vi "Create Tick Lines.vi"(0 "Grid Plane Visible":T1, 1 "Major Ticks":u16, 2 "Minor Ticks":u16, 3 "Major Color":u32(colorbox), 4 "Minor Color":u32(colorbox), 5 "error in (no error)":errorcluster, 6 "Tick Cluster Array":T2, 7 "Draw Major":bool, 8 "Range":cluster{"Max":sgl, "Min":sgl}, 9 "Draw Minor":bool, 10 "Axis":enum16{"X-Axis", "Y-Axis", "Z-Axis"}(ring), 11 "Inverted?":bool, 13 "Logarithm?":bool) -> (14 "Axis Tick Object Out":refnum<vi>, 19 "error out":errorcluster)   [LabVIEW 2020, in "3D Plot.lvclass"]
uses:
  <vilib>/Math Plots/3D Math Plots/3D Plot/3D Plot/3D Plot.lvclass
  <vilib>/Math Plots/3D Math Plots/3D Plot/3D Plot/Typedef/Tick Array.ctl
  <vilib>/picture/3D Picture Control/Object/Create Object (name).vi
  <vilib>/picture/3D Picture Control/NI_3D Picture Control.lvlib
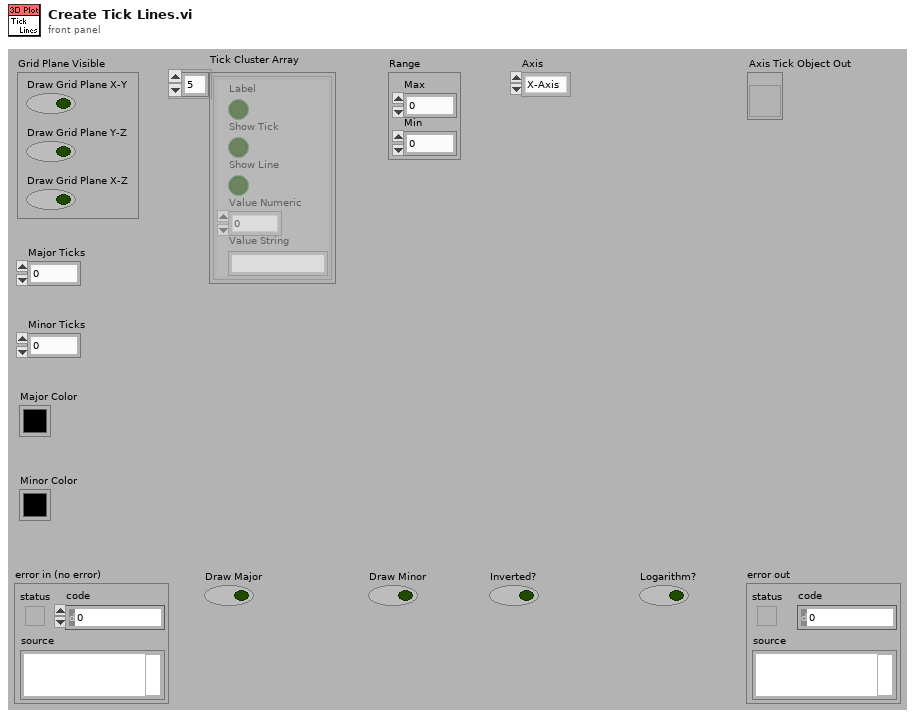
[diagram p1: front panel]
types:
  T1 = cluster{"Draw Grid Plane X-Y":bool, "Draw Grid Plane Y-Z":bool, "Draw Grid Plane X-Z":bool}
  T2 = typedef "3D Plot.lvclass/Tick Array.ctl" = cluster{"Label":bool, "Show Tick":bool, "Show Line":bool, "Value Numeric":sgl, "Value String":string}[]
  T3 = enum16{"Overall", "Per Primitive", "Per Vertex", "Binding Off"}
  T4 = enum16{"Points", "Lines", "Line Strip", "Line Loop", "Triangles", "Triangle Strip", "Triangle Fan", "Quads", "Quad Strip", "Polygon"}
  T5 = cluster{"length":sgl, "length":sgl, "length":sgl}
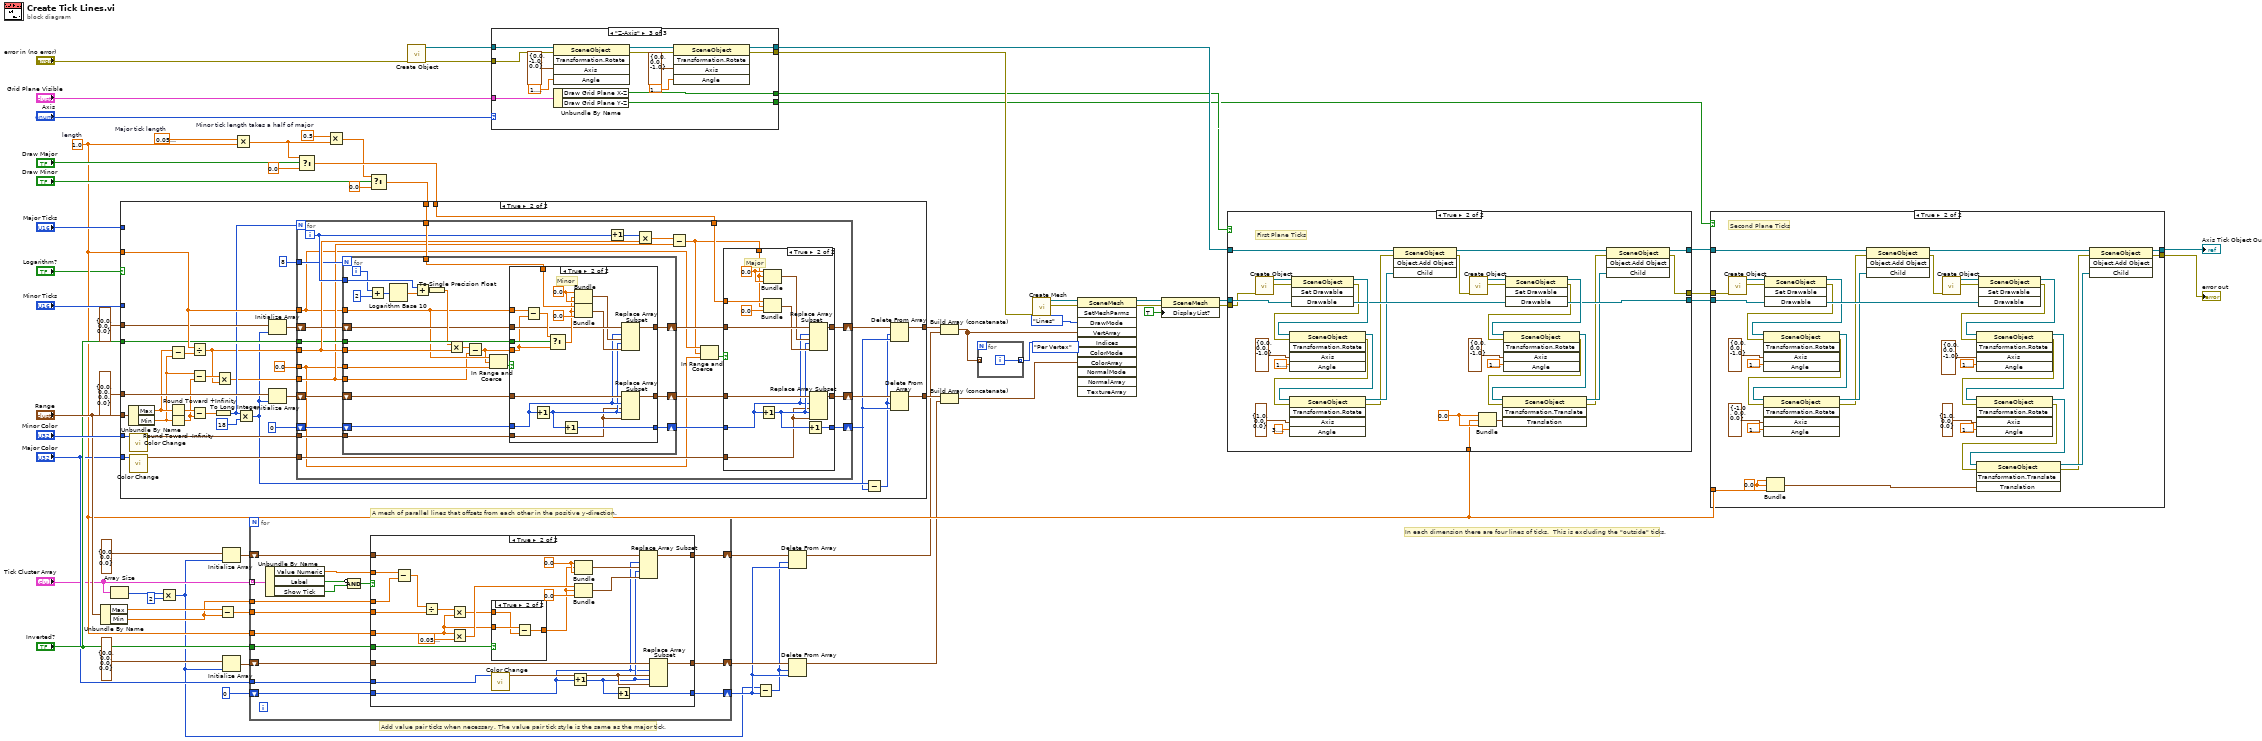
[diagram p0: block diagram]
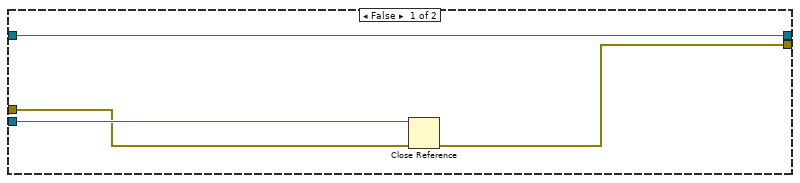
[diagram p2: hidden frame]
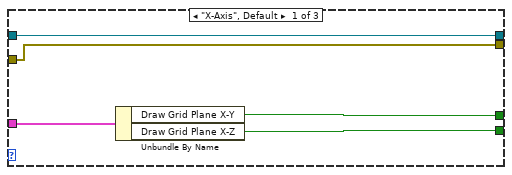
[diagram p4: hidden frame]
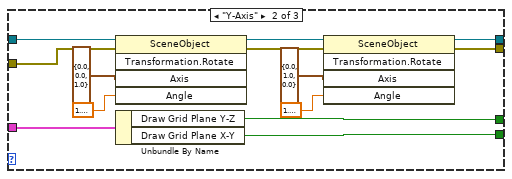
[diagram p5: hidden frame]
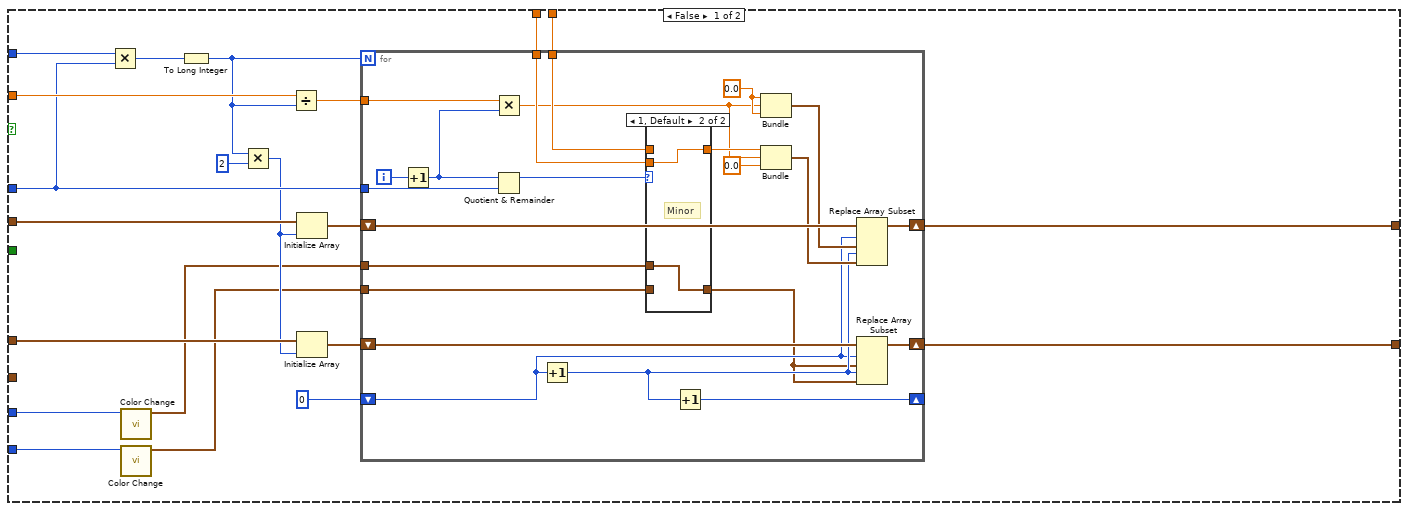
[diagram p6: hidden frame]
diagram:
  w57 = sgl 1.0  # length
  w39 = sgl 0.5  # Minor tick length takes a half of major
  w38 = sgl 0.05  # Major tick length
  # "Add value pair ticks when necessary. The value pair tick style is the same as the major tick."
  # "In each dimension there are four lines of ticks.  This is excluding the \"outside\" ticks."
  # "A mesh of parallel lines that offsets from each other in the positive y-direction."
  n1 = Unbundle By Name("Range") -> ("Max"=w25:sgl, "Min"=w24:sgl)
  n2 = Array Size(array="Tick Cluster Array") -> (size(s)=w4:i32)
  n3 = Multiply(x=w4, y=2 ("x")) -> (x*y=w2:i32)
  n4 = Subtract(x=w25, y=w24) -> (x-y=w35:sgl)
  n5 = Initialize Array(cluster{"X":sgl, "Y":sgl, "Z":sgl} {"X"=0.0, "Y"=0.0, "Z"=0.0} ("3D Point"), w2) -> (w13:cluster{"X":sgl, "Y":sgl, "Z":sgl}[])
  n6 = Initialize Array(cluster{"R":sgl, "G":sgl, "B":sgl, "A":sgl} {"R"=0.0, "G"=0.0, "B"=0.0, "A"=0.0} ("RGBA"), w2) -> (w11:cluster{"R":sgl, "G":sgl, "B":sgl, "A":sgl}[])
  n7 = Multiply(x=w38, y=w57) -> (x*y=w45:sgl)
  n8 = for {
    tunnel: "Tick Cluster Array" -> [w82] mode=indexing
    tunnel: w57 -> [w75]
    tunnel: w35 -> [w77]
    tunnel: w24 -> [w76]
    tunnel: "Inverted?" -> [w74]
    tunnel: "Major Color" -> [w73]
    shift-right: [w72] -> w7
    shift-left: w11 -> [w71]
    shift-right: [w70] -> w9
    shift-left: w13 -> [w69]
    shift-right: [w67] -> w5
    shift-left: 0 -> [w68]
    n9 = Unbundle By Name(w82) -> ("Value Numeric"=w78:sgl, "Label"=w81:bool, "Show Tick"=w80:bool)
    n10 = Compound Arithmetic op=AND(invert w81, w80) -> (w79:bool)
    n11 = case shown="True" w79 {
      tunnel: w78 -> [_ w104]
      tunnel: w77 -> [_ w108]
      tunnel: w76 -> [_ w107]
      tunnel: w75 -> [_ w97]
      tunnel: w74 -> [_ w99]
      tunnel: w73 -> [_ w102]
      tunnel: [w84 w89] -> w72
      tunnel: w71 -> [w84 w90]
      tunnel: [w85 w91] -> w70
      tunnel: w69 -> [w85 w94]
      tunnel: w68 -> [w83 w86]
      tunnel: [w83 w95] -> w67
      frame False {
      }
      frame True {
        w100 = sgl 0.0
        n12 = Subtract(x=w104, y=w107) -> (x-y=w106:sgl)
        n13 = Divide(x=w106, y=w108) -> (x/y=w105:sgl)
        n14 = Multiply(x=w105, y=w97) -> (x*y=w98:sgl)
        n15 = Multiply(x=w97, y=sgl 0.05 ("x")) -> (x*y=w103:sgl)
        n16 = case shown="True" w99 {
          tunnel: w98 -> [w110 w112]
          tunnel: w97 -> [_ w113]
          tunnel: [w110 w111] -> w96
          frame False {
          }
          frame True {
            n17 = Subtract(x=w113, y=w112) -> (x-y=w111:sgl)
          }
        }
        n18 = call <vilib>:"Color Change.vi"("Color"=w102) -> ("RGBA"=w88:cluster{"R":sgl, "G":sgl, "B":sgl, "A":sgl})  [unwired: 1 in, 9 out]
        n19 = Increment(x=w86) -> (x+1=w87:i32)
        n20 = Bundle(w100, w96, w100) -> (w93:cluster{sgl, sgl, sgl})  [unwired: 1 out]
        n21 = Bundle(w103, w96, sgl 0.0) -> (w92:cluster{sgl, sgl, sgl})  [unwired: 1 out]
        n22 = Increment(x=w87) -> (x+1=w95:i32)
        n23 = Replace Array Subset(array=w94, new element #1=w93, index #1=w86, new element #2=w92, index #2=w87) -> (w91:cluster{"X":sgl, "Y":sgl, "Z":sgl}[])
        n24 = Replace Array Subset(array=w90, new element #1=w88, index #1=w86, new element #2=w88, index #2=w87) -> (w89:cluster{"R":sgl, "G":sgl, "B":sgl, "A":sgl}[])
      }
    }
  }
  n25 = Select(t=w45, s="Draw Major", f=sgl 0.0) -> (s? t:f=w50:sgl)
  n26 = Multiply(x=w39, y=w45) -> (x*y=w48:sgl)
  n27 = Select(t=w48, s="Draw Minor", f=sgl 0.0) -> (s? t:f=w47:sgl)
  n28 = case shown="True" "Logarithm?" {
    tunnel: w50 -> [w134 w192]
    tunnel: w47 -> [w133 w193]
    tunnel: "Minor Color" -> [w115 w166]
    tunnel: cluster{"R":sgl, "G":sgl, "B":sgl, "A":sgl} {"R"=0.0, "G"=0.0, "B"=0.0, "A"=0.0} ("RGBA") -> [w125 w187]
    tunnel: "Major Color" -> [w117 w168]
    tunnel: w57 -> [w131 w191]
    tunnel: [w130 w171] -> w34
    tunnel: [w129 w169] -> w33
    tunnel: "Minor Ticks" -> [w128 _]
    tunnel: "Major Ticks" -> [w127 _]
    tunnel: "Range" -> [_ w195]
    tunnel: "Inverted?" -> [_ w190]
    tunnel: cluster{"X":sgl, "Y":sgl, "Z":sgl} {"X"=0.0, "Y"=0.0, "Z"=0.0} ("3D Point") -> [w126 w189]
    frame False {
      n29 = Multiply(x=w127, y=w128) -> (x*y=w122:u16)
      n30 = call <vilib>:"Color Change.vi"("Color"=w115) -> ("RGBA"=w114:cluster{"R":sgl, "G":sgl, "B":sgl, "A":sgl})  [unwired: 1 in, 9 out]
      n31 = call <vilib>:"Color Change.vi"("Color"=w117) -> ("RGBA"=w116:cluster{"R":sgl, "G":sgl, "B":sgl, "A":sgl})  [unwired: 1 in, 9 out]
      n32 = To Long Integer(number=w122) -> (32bit integer=w118:i32)
      n33 = Multiply(x=w118, y=2) -> (x*y=w120:i32)
      n34 = Divide(x=w131, y=w118) -> (x/y=w132:sgl)
      n35 = Initialize Array(w126, w120) -> (w123:cluster{"X":sgl, "Y":sgl, "Z":sgl}[])
      n36 = Initialize Array(w125, w120) -> (w124:cluster{"R":sgl, "G":sgl, "B":sgl, "A":sgl}[])
      n37 = for {
        N: w118 -> [_]
        tunnel: w132 -> [w157]
        tunnel: w128 -> [w156]
        tunnel: w134 -> [w155]
        tunnel: w133 -> [w154]
        shift-right: [w142] -> w130
        shift-left: w123 -> [w145]
        tunnel: w116 -> [w149]
        tunnel: w114 -> [w148]
        shift-right: [w140] -> w129
        shift-left: w124 -> [w141]
        shift-right: [w139] -> _
        shift-left: 0 ("y") -> [w137]
        i -> [w147]
        w146 = sgl 0.0
        n38 = Increment(x=w147) -> (x+1=w150:i32)
        n39 = Multiply(x=w157, y=w150) -> (x*y=w136:sgl)
        n40 = Quotient & Remainder(x=w150, y=w156) -> (x-y*floor(x/y)=w153:i32)  [unwired: 1 out]
        n41 = Increment(x=w137) -> (x+1=w138:i32)
        n42 = case shown="1, Default" w153 {
          tunnel: w155 -> [w159 _]
          tunnel: w154 -> [_ w161]
          tunnel: [w159 w161] -> w151
          tunnel: w149 -> [w158 _]
          tunnel: w148 -> [_ w160]
          tunnel: [w158 w160] -> w135
          frame 0 {
            # "Major"
          }
          frame 1, Default {
            # "Minor"
          }
        }
        n43 = Increment(x=w138) -> (x+1=w139:i32)
        n44 = Bundle(w146, w136, w146) -> (w144:cluster{sgl, sgl, sgl})  [unwired: 1 out]
        n45 = Bundle("f"=w151, w136, sgl 0.0) -> (w143:cluster{"f":sgl, sgl, sgl})  [unwired: 1 out]
        n46 = Replace Array Subset(array=w145, new element #1=w144, index #1=w137, new element #2=w143, index #2=w138) -> (w142:cluster{"X":sgl, "Y":sgl, "Z":sgl}[])
        n47 = Replace Array Subset(array=w141, new element #1=w135, index #1=w137, new element #2=w135, index #2=w138) -> (w140:cluster{"R":sgl, "G":sgl, "B":sgl, "A":sgl}[])
      }
    }
    frame True {
      n48 = Unbundle By Name(w195) -> ("Max"=w180:sgl, "Min"=w178:sgl)
      n49 = call <vilib>:"Color Change.vi"("Color"=w166) -> ("RGBA"=w165:cluster{"R":sgl, "G":sgl, "B":sgl, "A":sgl})  [unwired: 1 in, 9 out]
      n50 = call <vilib>:"Color Change.vi"("Color"=w168) -> ("RGBA"=w167:cluster{"R":sgl, "G":sgl, "B":sgl, "A":sgl})  [unwired: 1 in, 9 out]
      n51 = Subtract(x=w180, y=w178) -> (x-y=w179:sgl)
      n52 = Round Toward +Infinity(x=w180) -> (ceil(x): smallest int >= x=w181:sgl)
      n53 = Round Toward -Infinity(1:w178) -> (0:w177:sgl)
      n54 = Divide(x=w191, y=w179) -> (x/y=w175:sgl)
      n55 = Subtract(x=w178, y=w177) -> (x-y=w176:sgl)
      n56 = Subtract(x=w181, y=w177) -> (x-y=w194:sgl)
      n57 = To Long Integer(number=w194) -> (32bit integer=w182:i32)
      n58 = Multiply(x=w176, y=w175) -> (x*y=w174:sgl)
      n59 = Multiply(x=w182, y=18 ("x")) -> (x*y=w164:i32)
      n60 = Initialize Array(w189, w164) -> (w188:cluster{"X":sgl, "Y":sgl, "Z":sgl}[])
      n61 = Initialize Array(w187, w164) -> (w186:cluster{"R":sgl, "G":sgl, "B":sgl, "A":sgl}[])
      n62 = for {
        N: w182 -> [_]
        shift-right: [w212] -> w170
        shift-left: w186 -> [w218]
        shift-right: [w214] -> w172
        shift-left: w188 -> [w219]
        tunnel: w175 -> [w208]
        tunnel: w193 -> [w217]
        tunnel: w165 -> [w216]
        tunnel: w192 -> [w211]
        tunnel: w167 -> [w202]
        tunnel: w191 -> [w199]
        tunnel: w190 -> [w207]
        shift-right: [w205] -> w163
        shift-left: 0 -> [w206]
        tunnel: 8 -> [w203]
        tunnel: w174 -> [w201]
        tunnel: sgl 0.0 ("lower limit") -> [w200]
        i -> [w210]
        n63 = for {
          N: w203 -> [_]
          shift-right: [w247] -> w215
          shift-left: w219 -> [w248]
          shift-right: [w245] -> w213
          shift-left: w218 -> [w246]
          tunnel: w210 -> [w255]
          tunnel: w208 -> [w254]
          tunnel: w217 -> [w252]
          tunnel: w216 -> [w251]
          tunnel: w199 -> [w241]
          tunnel: w207 -> [w250]
          shift-right: [w244] -> w204
          shift-left: w206 -> [w243]
          tunnel: w201 -> [w239]
          tunnel: w200 -> [w242]
          i -> [w253]
          n64 = Add(x=w253, y=2 ("x")) -> (x+y=w256:i32)
          n65 = Logarithm Base 10(1:w256) -> (0:w257:dbl)
          n66 = Add(x=w255, y=w257) -> (x+y=w259:dbl)
          n67 = To Single Precision Float(number=w259) -> (single precision float=w249:sgl)
          n68 = Multiply(x=w249, y=w254) -> (x*y=w240:sgl)
          n69 = Subtract(x=w240, y=w239) -> (x-y=w238:sgl)
          n70 = In Range and Coerce(upper limit=w241, x=w238, lower limit=w242) -> (In Range?=w237:bool)  [unwired: 1 out]
          n71 = case shown="True" w237 {
            tunnel: w252 -> [_ w278]
            tunnel: w251 -> [_ w263]
            tunnel: w250 -> [_ w275]
            tunnel: w248 -> [w262 w274]
            tunnel: [w262 w271] -> w247
            tunnel: w246 -> [w261 w270]
            tunnel: [w261 w269] -> w245
            tunnel: [w260 w268] -> w244
            tunnel: w243 -> [w260 w267]
            tunnel: w241 -> [_ w265]
            tunnel: w238 -> [_ w264]
            frame False {
            }
            frame True {
              w279 = sgl 0.0
              # "Minor"
              n72 = Subtract(x=w265, y=w264) -> (x-y=w276:sgl)
              n73 = Increment(x=w267) -> (x+1=w266:i32)
              n74 = Select(t=w276, s=w275, f=w264) -> (s? t:f=w277:sgl)
              n75 = Increment(x=w266) -> (x+1=w268:i32)
              n76 = Bundle(w279, w277, w279) -> (w273:cluster{sgl, sgl, sgl})  [unwired: 1 out]
              n77 = Bundle("f"=w278, w277, sgl 0.0) -> (w272:cluster{"f":sgl, sgl, sgl})  [unwired: 1 out]
              n78 = Replace Array Subset(array=w274, new element #1=w273, index #1=w267, new element #2=w272, index #2=w266) -> (w271:cluster{"X":sgl, "Y":sgl, "Z":sgl}[])
              n79 = Replace Array Subset(array=w270, new element #1=w263, index #1=w267, new element #2=w263, index #2=w266) -> (w269:cluster{"R":sgl, "G":sgl, "B":sgl, "A":sgl}[])
            }
          }
        }
        n80 = Increment(x=w210) -> (x+1=w209:i32)
        n81 = Multiply(x=w209, y=w208) -> (x*y=w197:sgl)
        n82 = Subtract(x=w197, y=w201) -> (x-y=w196:sgl)
        n83 = In Range and Coerce(upper limit=w199, x=w196, lower limit=w200) -> (In Range?=w198:bool)  [unwired: 1 out]
        n84 = case shown="True" w198 {
          tunnel: w215 -> [w222 w236]
          tunnel: [w222 w235] -> w214
          tunnel: w213 -> [w221 w234]
          tunnel: [w221 w233] -> w212
          tunnel: w211 -> [_ w230]
          tunnel: w196 -> [_ w229]
          tunnel: [w220 w226] -> w205
          tunnel: w204 -> [w220 w224]
          tunnel: w202 -> [_ w223]
          frame False {
          }
          frame True {
            w232 = sgl 0.0
            # "Major"
            n85 = Increment(x=w224) -> (x+1=w225:i32)
            n86 = Bundle(w232, w229, w232) -> (w228:cluster{sgl, sgl, sgl})  [unwired: 1 out]
            n87 = Bundle("f"=w230, w229, sgl 0.0) -> (w227:cluster{"f":sgl, sgl, sgl})  [unwired: 1 out]
            n88 = Increment(x=w225) -> (x+1=w226:i32)
            n89 = Replace Array Subset(array=w236, new element #1=w228, index #1=w224, new element #2=w227, index #2=w225) -> (w235:cluster{"X":sgl, "Y":sgl, "Z":sgl}[])
            n90 = Replace Array Subset(array=w234, new element #1=w223, index #1=w224, new element #2=w223, index #2=w225) -> (w233:cluster{"R":sgl, "G":sgl, "B":sgl, "A":sgl}[])
          }
        }
      }
      n91 = Subtract(x=w164, y=w163) -> (x-y=w162:i32)
      n92 = Delete From Array(array=w172, length=w162, index=w163) -> (array with subset deleted=w171:cluster{"X":sgl, "Y":sgl, "Z":sgl}[])  [unwired: 1 out]
      n93 = Delete From Array(array=w170, length=w162, index=w163) -> (array with subset deleted=w169:cluster{"R":sgl, "G":sgl, "B":sgl, "A":sgl}[])  [unwired: 1 out]
    }
  }
  n94 = call-poly <vilib>:"Create Object.vi"("error in (no error)"="error in (no error)") -> ("error out"=w21:errorcluster, "Scene:New Object"=w22:refnum<vi>)  [unwired: 9 in]
  n95 = case shown="\"Z-Axis\"" "Axis" {
    tunnel: [w285 w289 w303] -> w20
    tunnel: w22 -> [w285 w292 w305]
    tunnel: [w284 w290 w304] -> w23
    tunnel: w21 -> [w284 w291 w302]
    tunnel: "Grid Plane Visible" -> [w283 w288 w301]
    tunnel: [w282 w287 w300] -> w17
    tunnel: [w281 w286 w299] -> w18
    frame "X-Axis", Default {
      n96 = Unbundle By Name(w283) -> ("Draw Grid Plane X-Y"=w281:bool, "Draw Grid Plane X-Z"=w282:bool)
    }
    frame "Y-Axis" {
      n97 = invoke class="SceneObject" method="Transformation.Rotate"(reference=w292, error in=w291, "Axis"=cluster{"X":sgl, "Y":sgl, "Z":sgl} {"X"=0.0, "Y"=0.0, "Z"=1.0}, "Angle"=1.5707963267948966) -> (reference out=w297:refnum<vi>, error out=w298:errorcluster)  [unwired: 1 in, 3 out]
      n98 = Unbundle By Name(w288) -> ("Draw Grid Plane Y-Z"=w286:bool, "Draw Grid Plane X-Y"=w287:bool)
      n99 = invoke class="SceneObject" method="Transformation.Rotate"(reference=w297, error in=w298, "Axis"=cluster{"X":sgl, "Y":sgl, "Z":sgl} {"X"=0.0, "Y"=1.0, "Z"=0.0}, "Angle"=1.5707963267948966) -> (reference out=w289:refnum<vi>, error out=w290:errorcluster)  [unwired: 1 in, 3 out]
    }
    frame "Z-Axis" {
      n100 = invoke class="SceneObject" method="Transformation.Rotate"(reference=w305, error in=w302, "Axis"=cluster{"X":sgl, "Y":sgl, "Z":sgl} {"X"=0.0, "Y"=-1.0, "Z"=0.0}, "Angle"=1.5707963267948966) -> (reference out=w306:refnum<vi>, error out=w311:errorcluster)  [unwired: 1 in, 3 out]
      n101 = Unbundle By Name(w301) -> ("Draw Grid Plane X-Z"=w299:bool, "Draw Grid Plane Y-Z"=w300:bool)
      n102 = invoke class="SceneObject" method="Transformation.Rotate"(reference=w306, error in=w311, "Axis"=cluster{"X":sgl, "Y":sgl, "Z":sgl} {"X"=0.0, "Y"=0.0, "Z"=-1.0}, "Angle"=1.5707963267948966) -> (reference out=w303:refnum<vi>, error out=w304:errorcluster)  [unwired: 1 in, 3 out]
    }
  }
  n103 = Subtract(x=w2, y=w5) -> (x-y=w3:i32)
  n104 = Delete From Array(array=w9, length=w3, index=w5) -> (array with subset deleted=w8:cluster{"X":sgl, "Y":sgl, "Z":sgl}[])  [unwired: 1 out]
  n105 = Delete From Array(array=w7, length=w3, index=w5) -> (array with subset deleted=w6:cluster{"R":sgl, "G":sgl, "B":sgl, "A":sgl}[])  [unwired: 1 out]
  n106 = Build Array (concatenate)(w34, w8) -> (w31:cluster{"X":sgl, "Y":sgl, "Z":sgl}[])
  n107 = Build Array (concatenate)(w33, w6) -> (w32:cluster{"R":sgl, "G":sgl, "B":sgl, "A":sgl}[])
  n108 = for {
    tunnel: w31 -> [_] mode=indexing
    tunnel: [w312] -> w30 mode=indexing
    i -> [w312]
  }
  n109 = call <vilib>:"Create Mesh.vi"("error in (no error)"=w23) -> ("error out"=w29:errorcluster, "New Mesh Refnum"=w40:refnum<vi>)  [unwired: 9 out]
  n110 = invoke class="SceneMesh" method="SetMeshParms"(reference=w40, error in=w29, "DrawMode"=T4."Lines" ("Draw Mode"), "VertArray"=w31, "Indices"=w30, "ColorMode"=T3."Per Vertex" ("Color Binding Mode"), "ColorArray"=w32) -> (reference out=w43:refnum<vi>, error out=w28:errorcluster)  [unwired: 4 in, 9 out]
  n111 = property class="SceneMesh"(reference=w43, error in=w28, "DisplayList?"=TRUE ("Use Display List?")) -> (reference out=w36:refnum<vi>, error out=w27:errorcluster)
  n112 = case shown="True" w18 {
    tunnel: [w314 w344] -> w37
    tunnel: w36 -> [w314 w334]
    tunnel: w57 -> [_ w332]
    tunnel: w27 -> [w313 w331]
    tunnel: [w313 w317] -> w26
    tunnel: w20 -> [w315 w321]
    tunnel: [w315 w316] -> w19
    frame False {
    }
    frame True {
      w333 = sgl 0.0 ("length")
      # "First Plane Ticks"
      n113 = call-poly <vilib>:"Create Object.vi"("error in (no error)"=w331) -> ("error out"=w330:errorcluster, "Scene:New Object"=w349:refnum<vi>)  [unwired: 9 in]
      n114 = invoke class="SceneObject" method="Set Drawable"(reference=w349, error in=w330, "Drawable"=w334) -> (reference out=w348:refnum<vi>, error out=w329:errorcluster, "Drawable"=w345:refnum<vi>)  [unwired: 1 in, 1 out]
      n115 = invoke class="SceneObject" method="Transformation.Rotate"(reference=w348, error in=w329, "Axis"=cluster{"X":sgl, "Y":sgl, "Z":sgl} {"X"=0.0, "Y"=0.0, "Z"=-1.0}, "Angle"=sgl 1.5707964) -> (reference out=w343:refnum<vi>, error out=w328:errorcluster)  [unwired: 1 in, 3 out]
      n116 = invoke class="SceneObject" method="Transformation.Rotate"(reference=w343, error in=w328, "Axis"=cluster{"X":sgl, "Y":sgl, "Z":sgl} {"X"=1.0, "Y"=0.0, "Z"=0.0}, "Angle"=sgl 3.1415927 ("length")) -> (reference out=w324:refnum<vi>, error out=w323:errorcluster)  [unwired: 1 in, 3 out]
      n117 = invoke class="SceneObject" method="Object.Add Object"(reference=w321, error in=w323, "Child"=w324) -> (reference out=w320:refnum<vi>, error out=w322:errorcluster)  [unwired: 1 in, 2 out]
      n118 = call-poly <vilib>:"Create Object.vi"("error in (no error)"=w322) -> ("error out"=w327:errorcluster, "Scene:New Object"=w347:refnum<vi>)  [unwired: 9 in]
      n119 = Bundle("length"=w333, "length"=w332, "length"=w333) -> (w337:T5)  [unwired: 1 out]
      n120 = invoke class="SceneObject" method="Set Drawable"(reference=w347, error in=w327, "Drawable"=w345) -> (reference out=w346:refnum<vi>, error out=w326:errorcluster, "Drawable"=w344:refnum<vi>)  [unwired: 1 in, 1 out]
      n121 = invoke class="SceneObject" method="Transformation.Rotate"(reference=w346, error in=w326, "Axis"=cluster{"X":sgl, "Y":sgl, "Z":sgl} {"X"=0.0, "Y"=0.0, "Z"=-1.0}, "Angle"=sgl 1.5707964) -> (reference out=w338:refnum<vi>, error out=w325:errorcluster)  [unwired: 1 in, 3 out]
      n122 = invoke class="SceneObject" method="Transformation.Translate"(reference=w338, error in=w325, "Translation"=w337) -> (reference out=w319:refnum<vi>, error out=w318:errorcluster)  [unwired: 1 in, 2 out]
      n123 = invoke class="SceneObject" method="Object.Add Object"(reference=w320, error in=w318, "Child"=w319) -> (reference out=w316:refnum<vi>, error out=w317:errorcluster)  [unwired: 1 in, 2 out]
    }
  }
  n124 = case shown="True" w17 {
    tunnel: w37 -> [w352 w389]
    tunnel: w57 -> [_ w371]
    tunnel: w26 -> [w351 w363]
    tunnel: w19 -> [w353 w360]
    tunnel: [w353 w357] -> w62
    tunnel: [w350 w354] -> w56
    frame False {
      n125 = Close Reference(reference=w352, error in (no error)=w351) -> (error out=w350:errorcluster)
    }
    frame True {
      w372 = sgl 0.0 ("length")
      # "Second Plane Ticks"
      n126 = call-poly <vilib>:"Create Object.vi"("error in (no error)"=w363) -> ("error out"=w370:errorcluster, "Scene:New Object"=w390:refnum<vi>)  [unwired: 9 in]
      n127 = invoke class="SceneObject" method="Set Drawable"(reference=w390, error in=w370, "Drawable"=w389) -> (reference out=w373:refnum<vi>, error out=w369:errorcluster, "Drawable"=w387:refnum<vi>)  [unwired: 1 in, 1 out]
      n128 = invoke class="SceneObject" method="Transformation.Rotate"(reference=w373, error in=w369, "Axis"=cluster{"X":sgl, "Y":sgl, "Z":sgl} {"X"=0.0, "Y"=0.0, "Z"=-1.0}, "Angle"=sgl 1.5707964) -> (reference out=w381:refnum<vi>, error out=w368:errorcluster)  [unwired: 1 in, 3 out]
      n129 = invoke class="SceneObject" method="Transformation.Rotate"(reference=w381, error in=w368, "Axis"=cluster{"X":sgl, "Y":sgl, "Z":sgl} {"X"=-1.0, "Y"=0.0, "Z"=0.0}, "Angle"=sgl 1.5707964) -> (reference out=w361:refnum<vi>, error out=w359:errorcluster)  [unwired: 1 in, 3 out]
      n130 = Bundle("length"=w372, "length"=w372, "length"=w371) -> (w374:T5)  [unwired: 1 out]
      n131 = invoke class="SceneObject" method="Object.Add Object"(reference=w360, error in=w359, "Child"=w361) -> (reference out=w362:refnum<vi>, error out=w358:errorcluster)  [unwired: 1 in, 2 out]
      n132 = call-poly <vilib>:"Create Object.vi"("error in (no error)"=w358) -> ("error out"=w367:errorcluster, "Scene:New Object"=w388:refnum<vi>)  [unwired: 9 in]
      n133 = invoke class="SceneObject" method="Set Drawable"(reference=w388, error in=w367, "Drawable"=w387) -> (reference out=w386:refnum<vi>, error out=w366:errorcluster)  [unwired: 1 in, 2 out]
      n134 = invoke class="SceneObject" method="Transformation.Rotate"(reference=w386, error in=w366, "Axis"=cluster{"X":sgl, "Y":sgl, "Z":sgl} {"X"=0.0, "Y"=0.0, "Z"=-1.0}, "Angle"=sgl 1.5707964) -> (reference out=w380:refnum<vi>, error out=w365:errorcluster)  [unwired: 1 in, 3 out]
      n135 = invoke class="SceneObject" method="Transformation.Rotate"(reference=w380, error in=w365, "Axis"=cluster{"X":sgl, "Y":sgl, "Z":sgl} {"X"=1.0, "Y"=0.0, "Z"=0.0}, "Angle"=sgl 1.5707964) -> (reference out=w379:refnum<vi>, error out=w364:errorcluster)  [unwired: 1 in, 3 out]
      n136 = invoke class="SceneObject" method="Transformation.Translate"(reference=w379, error in=w364, "Translation"=w374) -> (reference out=w356:refnum<vi>, error out=w355:errorcluster)  [unwired: 1 in, 2 out]
      n137 = invoke class="SceneObject" method="Object.Add Object"(reference=w362, error in=w355, "Child"=w356) -> (reference out=w357:refnum<vi>, error out=w354:errorcluster)  [unwired: 1 in, 2 out]
    }
  }
  "error out" <- w56
  "Axis Tick Object Out" <- w62
